vi "Read Optimization Path.vi"(8 "error in":errorcluster, 11 "EMS Generic in":refnum<class "EMS Generic.lvclass">) -> (0 "error out":errorcluster, 2 "Optimization Relative Path":string, 3 "EMS Generic out":refnum<class "EMS Generic.lvclass">)   [LabVIEW 2018, in "EMS Generic Actor.lvlib" / "EMS Generic.lvclass"]
uses:
  EMS Generic.lvclass
  EMS Generic.lvclass/EMS Generic.ctl
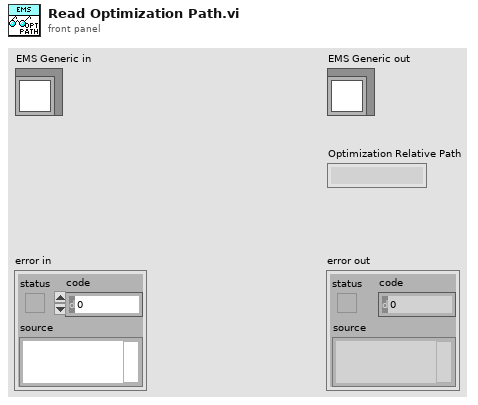
[diagram p1: front panel]
types:
  T1 = typedef "EMS Generic Actor.lvlib/EMS Generic.lvclass/Global Configuration.ctl" = cluster{"Microgrid ID":u8, "VF Device ID":T2, "Ongrid VF Priority":T2[], "Offgrid VF Priority":T2[], "AutoSwap Offgrid VF":u32, "AutoSwap Offgrid VF Delay (sec)":dbl, "AutoSwap Resynch VF":u32, "PCC Device ID":T2, "Device ID Array":T2[], "Nominal Voltage":dbl, "Nominal Frequency":dbl, "Resynch Timeout (sec)":dbl, "Island VF Activate Timeout (sec)":dbl, "Island PCC Target Power (kW)":dbl, "Island PCC Target Power Timeout (sec)":dbl, "Island Grid Settle Time (sec)":dbl, "Island PCC Failure Timeout (sec)":dbl, "Activation Devices Present Timeout (sec)":dbl, "Activation Devices Activated Timeout (sec)":dbl, "Blackstart VF GenMode Wait (sec)":dbl, "Blackstart VF DERCtrl Wait (sec)":dbl, "Blackstart Success Wait (sec)":dbl, "OnGrid Optimization Delay (sec)":dbl, "OffGrid Optimization Delay (sec)":dbl, "Resynch Frequency (Hz)":dbl, "Optimization Path":string}
  T2 = typedef "CSEISMIC DDS.lvlib/CSEISMIC DDS.lvclass/DeviceID.ctl" = string
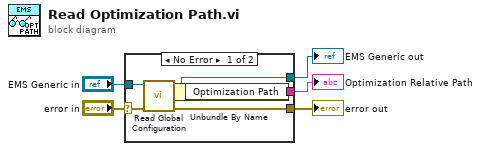
[diagram p0: block diagram]
diagram:
  n1 = case shown="No Error" "error in" {
    selector: "error in" -> [w9 w13]
    tunnel: [w8 w13] -> w3
    tunnel: [w10 w12] -> w1
    tunnel: "EMS Generic in" -> [w11 w12]
    tunnel: [w6 _] -> w2
    frame No Error {
      n2 = call "Read Global Configuration.vi"("error in"=w9, "EMS Generic in"=w11) -> ("error out"=w8:errorcluster, "Global Configuration"=w7:T1, "dup EMS Generic out"=w10:refnum<class "EMS Generic.lvclass">)  [unwired: 7 in]
      n3 = Unbundle By Name(w7) -> ("Optimization Path"=w6:string)
    }
    frame Error {
    }
  }
  "error out" <- w3
  "EMS Generic out" <- w1
  "Optimization Relative Path" <- w2
